vi "Align3DPointSetToPlaneXY.vi"(8 "error in":errorcluster, 11 "Point Set":T1[](array[typedef])) -> (0 "error out":errorcluster, 3 "Points Aligned to Plane":T1[](array[typedef]))   [LabVIEW 2020, in "ar.lvlib"]
doc: "Align 3D Points to a plane computed based on a Least Mean Squares plane-finding algorithm."
uses:
  ar.lvlib
  Plane Coefficients.ctl
  common/Object Point (Float).ctl
  common/common.lvlib
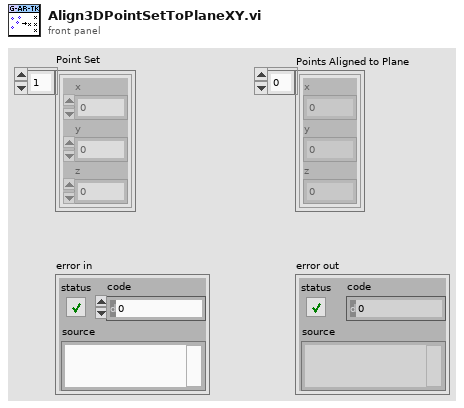
[diagram p1: front panel]
types:
  T1 = typedef "common.lvlib/Object Point (Float).ctl" = cluster{"x":dbl, "y":dbl, "z":dbl}
  T2 = typedef "ar.lvlib/Plane Coefficients.ctl" = cluster{"a":dbl, "b":dbl, "c":dbl, "d":dbl}
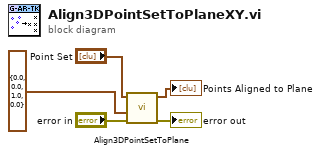
[diagram p0: block diagram]
diagram:
  n1 = call "Align3DPointSetToPlane.vi"("error in"="error in", "Plane Coefficients"=T2 {"a"=0.0, "b"=0.0, "c"=1.0, "d"=0.0} ("Plane Coeffcients"), "Point Set"="Point Set") -> ("error out"=→"error out":errorcluster, "Points Fitted to Plane"=→"Points Aligned to Plane":T1[])  [unwired: 7 in]
